vi "Get Object Item by Path (poly).vi"   [LabVIEW 2013, in "JSONtext.lvlib"]
uses:
  JSONtext.lvlib
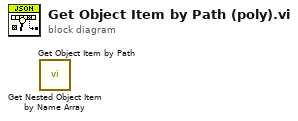
[diagram p0: block diagram]
diagram:
  n1 = call "Get Nested Object Item by Name Array.vi"() -> ()  [unwired: 8 in, 4 out]
  n2 = call "Get Object Item by Path.vi"() -> ()  [unwired: 8 in, 4 out]
